vi "checkInitialPosition.vi"(7 "Last mov.":u16(ring)=3 items=["unknown", "homing", "toLeft", "toRight"], 8 "error in (no error)":errorcluster, 9 "Step":dbl=0.1, 10 "Initial pos":dbl, 11 "Current pos":dbl) -> (0 "error out":errorcluster, 2 "go":bool=TRUE)   [LabVIEW 2023]
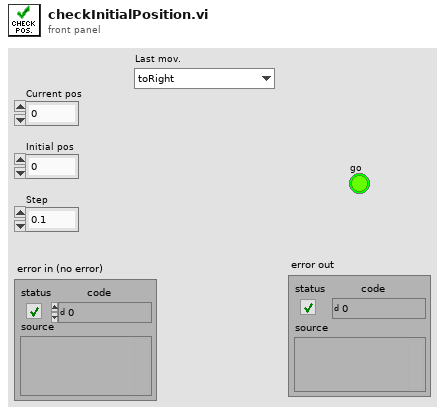
[diagram p1: front panel]
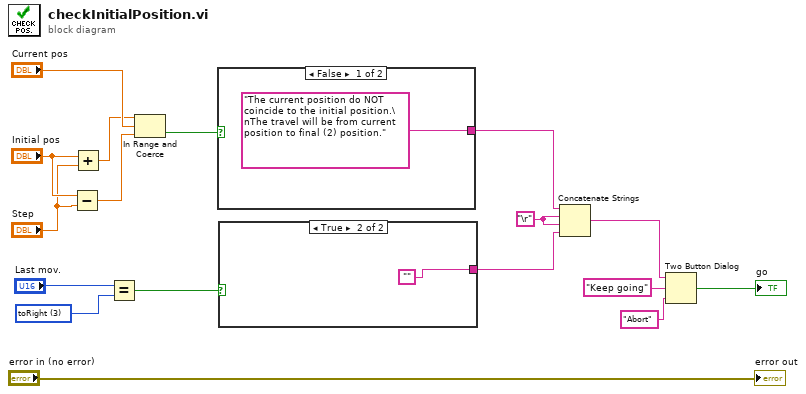
[diagram p0: block diagram]
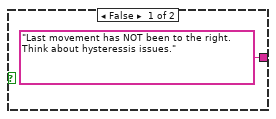
[diagram p2: hidden frame]
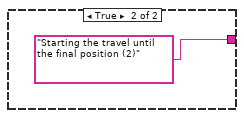
[diagram p3: hidden frame]
diagram:
  w4 = "\r"
  w7 = u16 3 items=["unknown", "homing", "toLeft", "toRight"] ("Last mov.")
  n1 = Subtract(x="Initial pos", y="Step") -> (x-y=w11:dbl)
  n2 = Add(x="Initial pos", y="Step") -> (x+y=w12:dbl)
  n3 = Equal?(x="Last mov.", y=w7) -> (x = y?=w5:bool)
  n4 = In Range and Coerce(upper limit=w12, x="Current pos", lower limit=w11) -> (In Range?=w6:bool)  [unwired: 1 out]
  n5 = case shown="False" w6 {
    tunnel: ["The current position do NOT coincide to the initial position.\nThe travel will be from current position to final (2) position." "Starting the travel until the final position (2)"] -> w3
    frame False {
    }
    frame True {
    }
  }
  n6 = case shown="True" w5 {
    tunnel: ["Last movement has NOT been to the right. Think about hysteressis issues." ""] -> w2
    frame False {
    }
    frame True {
    }
  }
  n7 = Concatenate Strings(w3, w4, w4, w2) -> (w1:string)
  n8 = Two Button Dialog(message=w1, 1:"Abort" ("F button name (\"Cancel\")"), 2:"Keep going" ("T button name (\"OK\")")) -> (T button?=→"go":bool)
  "error out" <- "error in (no error)"
